vi "MainDyno.vi"() -> ()   [LabVIEW 2017]
uses:
  <vilib>/DAQmx/read.llb/DAQmx Read (Analog 1D Wfm NChan NSamp).vi
  <vilib>/DAQmx/write.llb/DAQmx Write (Analog Wfm 1Chan NSamp).vi
  <vilib>/DAQmx/read.llb/DAQmx Read (Counter 1D DBL 1Chan NSamp).vi
  <vilib>/DAQmx/write.llb/DAQmx Write (Digital Bool 1Line 1Point).vi
  <vilib>/Analysis/baseanly.llb/Mean (DBL).vi
  <vilib>/DAQmx/miscellaneous.llb/DAQmx Fill In Error Info.vi
  <vilib>/Analysis/NI_AALBase.lvlib
  <vilib>/measure/NI_MABase.lvlib
  <resource>/objmgr/daqmx.rc
panel:
  out "XY Graph":cluster{dbl[], dbl[]}(graph)
  out "Array":dbl[](array[numeric])
  out "Waveform Graph 2":waveform(dbl)(graph)
  out "mean":dbl format="%0.2f"
  out "Waveform Graph":waveform(dbl)(graph)
  in  "VOUT":dbl(knob) scale=0.0..10.0
  in  "Boolean":bool
  in  "stop":bool
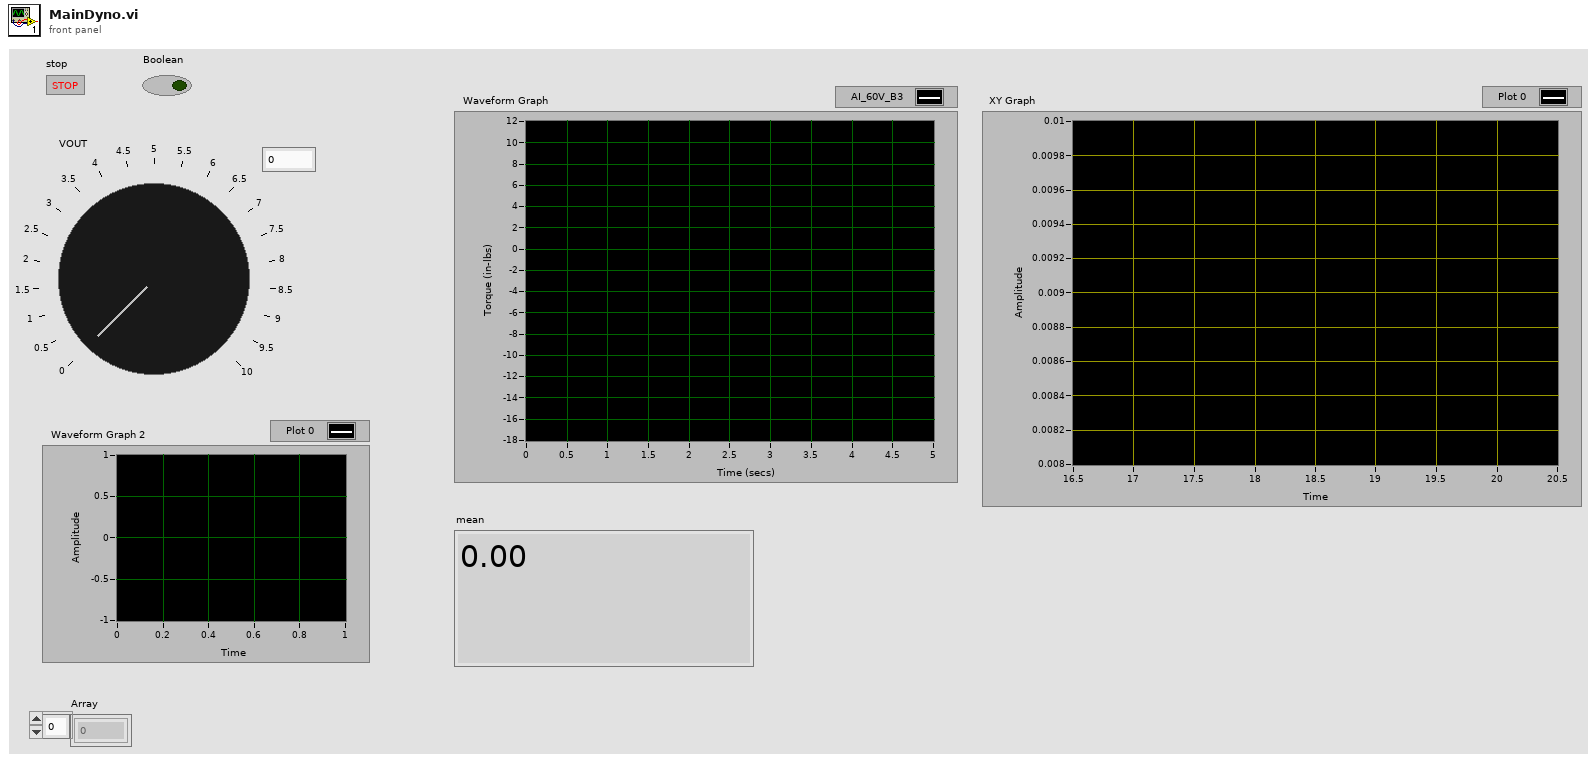
[diagram p1: front panel]
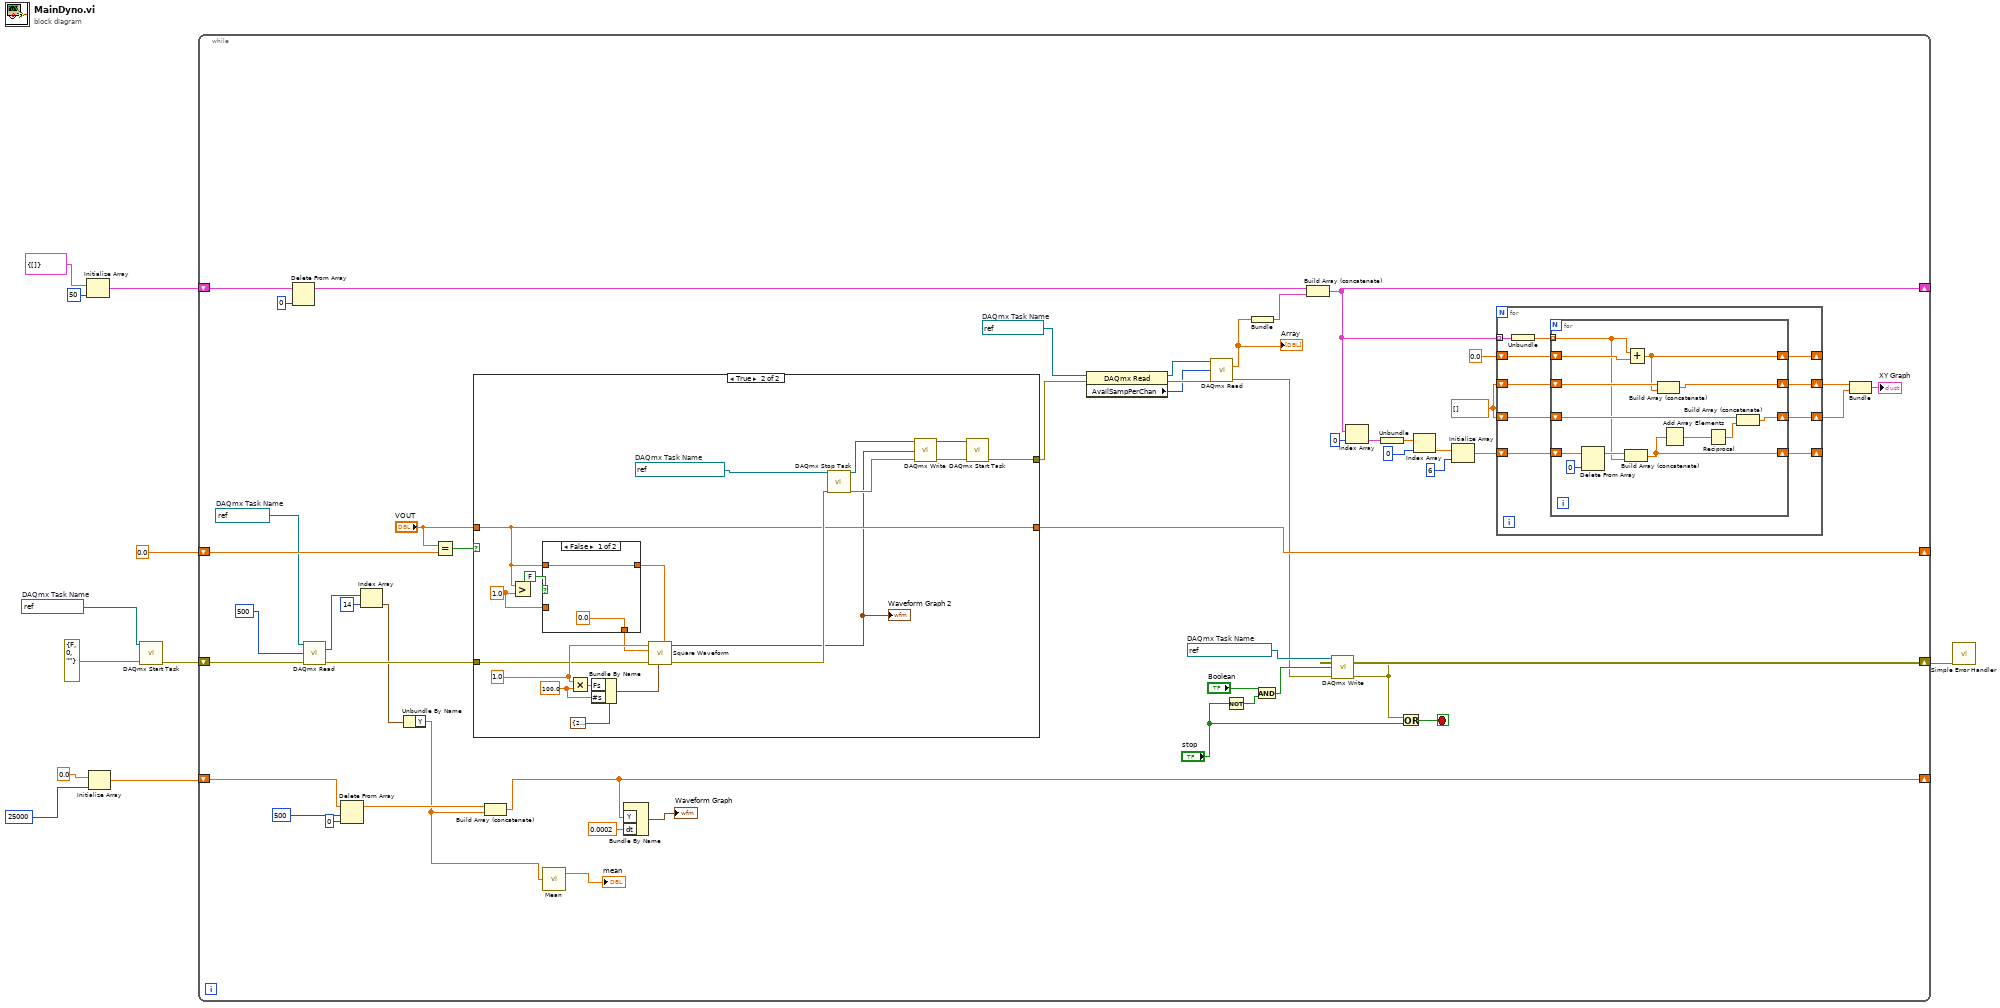
[diagram p0: block diagram]
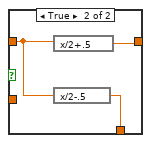
[diagram p3: hidden frame]
diagram:
  w4 = refnum<k21> "PrecorCTR"  # DAQmx Task Name
  n1 = Initialize Array(cluster{dbl[]} {[]}, 50 ("dimension size")) -> (w3:cluster{dbl[]}[])
  n2 = Initialize Array(0.0, 25000 ("dimension size")) -> (w9:dbl[])
  n3 = call <vilib>:"DAQmx Start Task.vi"("task/channels in"=w4, "error in"=errorcluster {"status"=FALSE, "code"=0, "source"=""} ("error constant")) -> ("error out"=w6:errorcluster)  [unwired: 12 in, 1 out]
  n4 = while {
    shift-right: [w61] -> w11
    shift-left: w6 -> [w56]
    shift-right: [w57] -> _
    shift-left: 0.0 -> [w60]
    shift-right: [w41] -> _
    shift-left: w9 -> [w45]
    shift-right: [w19] -> _
    shift-left: w3 -> [w29]
    stop <- w62 stop-if-true
    w23 = dbl[] []
    w34 = refnum<k21> "PrecorCTR"  # DAQmx Task Name
    w36 = refnum<k21> "PrecorMCEnable"  # DAQmx Task Name
    w37 = refnum<k21> "PrecorAI"  # DAQmx Task Name
    n5 = Delete From Array(array=w29, index=0) -> (array with subset deleted=w26:cluster{dbl[]}[])  [unwired: 1 in, 1 out]
    n6 = call-poly <vilib>:"DAQmx Read.vi"("task/channels in"=w37, "number of samples per channel"=500, "error in"=w56) -> ("data"=w53:waveform(dbl)[], "error out"=w55:errorcluster)  [unwired: 10 in, 1 out]
    n7 = Delete From Array(array=w45, length=500, index=0) -> (array with subset deleted=w43:dbl[])  [unwired: 1 out]
    n8 = Index Array(array=w53, index=14) -> (element=w47:waveform(dbl))
    n9 = Unbundle By Name(w47) -> ("Y"=w38:dbl[])
    n10 = Equal?(x="VOUT", y=w60) -> (x = y?=w59:bool)
    n11 = case shown="True" w59 {
      tunnel: "VOUT" -> [w87 w93]
      tunnel: w55 -> [w86 w97]
      tunnel: [w86 w104] -> w33
      tunnel: [w87 w93] -> w57
      frame False {
      }
      frame True {
        w88 = refnum<k21> "PrecorPulsedRPM"  # DAQmx Task Name
        w91 = 1.0 ("y")
        w98 = 1.0
        w101 = 100.0 ("y")
        n12 = Greater?(x=w93, y=w91) -> ()  [unwired: 1 out]
        n13 = case shown="False" FALSE {
          tunnel: [0.0 w110] -> w94
          tunnel: w93 -> [w107 w109]
          tunnel: [w107 w111] -> w92
          tunnel: w91 -> [_ _]
          frame False {
          }
          frame True {
            n14 = expression code="x/2+.5"(w109) -> (w111:dbl)
            n15 = expression code="x/2-.5"(w109) -> (w110:dbl)
          }
        }
        n16 = Multiply(x=w98, y=w101) -> (x*y=w102:dbl)
        n17 = Bundle By Name(cluster=cluster{"Fs":dbl, "#s":dbl} {"Fs"=20.0, "#s"=20.0} ("sampling info"), "Fs"=w102, "#s"=w101) -> (w95:cluster{"Fs":dbl, "#s":dbl})
        n18 = call <vilib>:"Square Waveform.vi"("offset"=w92, "sampling info"=w95, "error in (no error)"=w97, "amplitude"=w94, "frequency"=w98) -> ("error out"=w96:errorcluster, "signal out"=w90:waveform(dbl))  [unwired: 5 in]
        "Waveform Graph 2" <- w90
        n19 = call <vilib>:"DAQmx Stop Task.vi"("task/channels in"=w88, "error in"=w96) -> ("task out"=w100:refnum<k21>, "error out"=w99:errorcluster)  [unwired: 12 in]
        n20 = call-poly <vilib>:"DAQmx Write.vi"("task/channels in"=w100, "data"=w90, "error in"=w99) -> ("task out"=w106:refnum<k21>, "error out"=w105:errorcluster)  [unwired: 10 in, 1 out]
        n21 = call <vilib>:"DAQmx Start Task.vi"("task/channels in"=w106, "error in"=w105) -> ("error out"=w104:errorcluster)  [unwired: 12 in, 1 out]
      }
    }
    n22 = Build Array (concatenate)(w43, w38) -> (w41:dbl[])
    n23 = call-poly <vilib>:"Mean.vi"("X"=w38) -> ("mean"=→"mean":dbl)  [unwired: 1 out]
    n24 = Bundle By Name("Y"=w41, "dt"=0.0002) -> (→"Waveform Graph":waveform(dbl))  [unwired: 1 in]
    n25 = property class="DAQmx Read"(reference=w34, error in=w33) -> (reference out=w32:refnum<k21>, error out=w31:errorcluster, "AvailSampPerChan"=w30:u32)
    n26 = call-poly <vilib>:"DAQmx Read.vi"("task/channels in"=w32, "number of samples per channel"=w30, "error in"=w31) -> ("data"=w27:dbl[], "error out"=w35:errorcluster)  [unwired: 10 in, 1 out]
    "Array" <- w27
    n27 = Not(x="stop") -> (.not. x?=w49:bool)
    n28 = Bundle("data"=w27) -> (w25:cluster{"data":dbl[]})  [unwired: 1 in]
    n29 = And(x="Boolean", y=w49) -> (x .and. y?=w48:bool)
    n30 = Build Array (concatenate)(w26, w25) -> (w19:cluster{"data":dbl[]}[])
    n31 = call-poly <vilib>:"DAQmx Write.vi"("task/channels in"=w36, "data"=w48, "error in"=w35) -> ("error out"=w61:errorcluster)  [unwired: 10 in, 2 out]
    n32 = Index Array(array=w19, index=0) -> (element=w17:cluster{"data":dbl[]})
    n33 = Unbundle(w17) -> ("data"=w16:dbl[])
    n34 = Or(x=w61, y="stop") -> (x .or. y?=w62:bool)
    n35 = Index Array(array=w16, index=0) -> (element=w14:dbl)
    n36 = Initialize Array(w14, 6 ("dimension size")) -> (w12:dbl[])
    n37 = for {
      tunnel: w19 -> [w72] mode=indexing
      shift-right: [w66] -> w22
      shift-left: w23 -> [w70]
      shift-right: [w65] -> w21
      shift-left: w23 -> [w69]
      shift-right: [w67] -> _
      shift-left: 0.0 -> [w68]
      shift-right: [w63] -> _
      shift-left: w12 -> [w64]
      n38 = Unbundle(w72) -> ("data"=w71:dbl[])
      n39 = for {
        tunnel: w71 -> [w75] mode=indexing
        shift-right: [w82] -> w66
        shift-left: w70 -> [w85]
        shift-right: [w80] -> w65
        shift-left: w69 -> [w81]
        shift-right: [w83] -> w67
        shift-left: w68 -> [w84]
        shift-right: [w73] -> w63
        shift-left: w64 -> [w78]
        n40 = Delete From Array(array=w78, index=0) -> (array with subset deleted=w76:dbl[])  [unwired: 1 in, 1 out]
        n41 = Build Array (concatenate)(w76, w75) -> (w73:dbl[])
        n42 = Add(x=w75, y=w84) -> (x+y=w83:dbl)
        n43 = Build Array (concatenate)(w85, w83) -> (w82:dbl[])
        n44 = Add Array Elements(numeric array=w73) -> (sum=w74:dbl)
        n45 = Reciprocal(x=w74) -> (1/x=w79:dbl)
        n46 = Build Array (concatenate)(w81, w79) -> (w80:dbl[])
      }
    }
    n47 = Bundle(w22, w21) -> (→"XY Graph":cluster{dbl[], dbl[]})  [unwired: 1 in]
  }
  n48 = call <vilib>:"Simple Error Handler.vi"("error in (no error)"=w11) -> ()  [unwired: 4 in, 5 out]
